vi "convert to binary.vi"() -> ()   [LabVIEW 2018]
panel:
  out "reversed array":dbl[](array[numeric])
  in  "Numeric":dbl
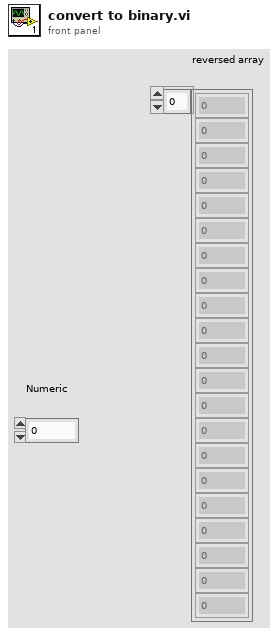
[diagram p1: front panel]
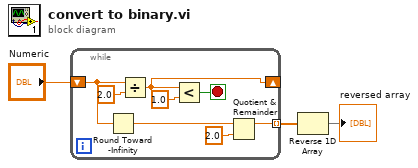
[diagram p0: block diagram]
diagram:
  n1 = while {
    tunnel: [w8] -> w2 mode=indexing
    shift-right: [w6] -> _
    shift-left: "Numeric" -> [w4]
    stop <- w10 stop-if-true
    n2 = Round Toward -Infinity(1:w4) -> (0:w5:dbl)
    n3 = Divide(x=w4, y=2.0) -> (x/y=w6:dbl)
    n4 = Less?(x=w6, y=1.0) -> (x < y?=w10:bool)
    n5 = Quotient & Remainder(x=w5, y=2.0) -> (x-y*floor(x/y)=w8:dbl)  [unwired: 1 out]
  }
  n6 = Reverse 1D Array(array=w2) -> (reversed array=→"reversed array":dbl[])
